vi "Filter Error Terms.vi"(11 "Terms[]":refnum<vi>[](array[refnum])) -> (3 "Terms[] out":refnum<vi>[](array[refnum]))   [LabVIEW 2017, in "CSM-Helper.lvclass"]
uses:
  CSM-Helper.lvclass
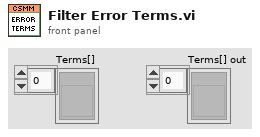
[diagram p1: front panel]
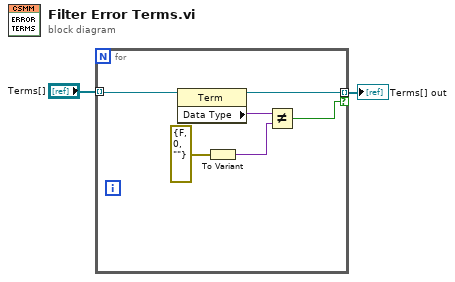
[diagram p0: block diagram]
diagram:
  n1 = for {
    tunnel: "Terms[]" -> [w8] mode=indexing
    tunnel: [w7] -> w1 mode=indexing if=w3
    n2 = property class="Term"(reference=w8) -> (reference out=w7:refnum<vi>, "Data Type"=w6:variant)  [unwired: 1 in, 1 out]
    n3 = To Variant(anything=errorcluster {"status"=FALSE, "code"=0, "source"=""} ("error in (no error)")) -> (Variant=w4:variant)
    n4 = Not Equal?(x=w6, y=w4) -> (x != y?=w3:bool)
  }
  "Terms[] out" <- w1
